vi "LogToDashboard.vi"(8 "error in (no error)":errorcluster, 11 "Info":string) -> (0 "error out":errorcluster)   [LabVIEW 2012]
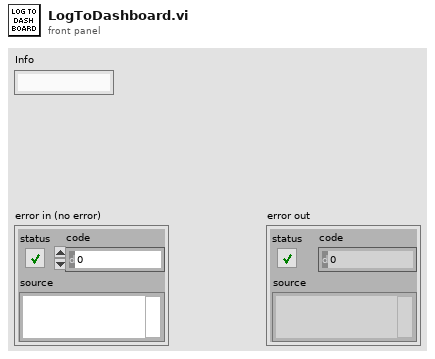
[diagram p1: front panel]
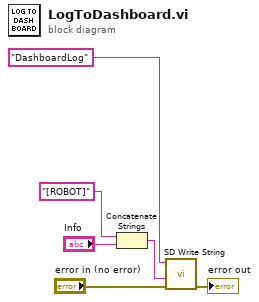
[diagram p0: block diagram]
diagram:
  n1 = Concatenate Strings("[ROBOT]" ("string"), "Info") -> (w4:string)
  n2 = call <vilib>:"SD Write String.vi"("error in"="error in (no error)", "String"=w4, "Name"="DashboardLog" ("format string")) -> ("error out"=→"error out":errorcluster)  [unwired: 7 in, 1 out]
